vi "CompleteResourceUtilizationWithIFw.vi"() -> ()   [LabVIEW 2015]
uses:
  <instrlib>/_niInstr/PIO Register Bus/v0/Common/Command From Host.ctl
  <vilib>/Platform/TimedLoop/XDataNode/timing_clust.ctl
  <vilib>/Platform/TimedLoop/XDataNode/nitl_modes.ctl
  <vilib>/Platform/TimedLoop/XDataNode/wakeup.ctl
  <vilib>/rvi/Emulation/niFpgaGetClockAttributes.vi
  <vilib>/rvi/Emulation/niFpgaSctlEmulationGetInTimedLoop.vi
  <vilib>/rvi/Emulation/niFpgaEmulationReportErrorSimple.vi
  <vilib>/rvi/eio/common/nirviEmuTemplateMethod_errors.vi
  <vilib>/rvi/Emulation/niFpgaCriticalErrorInLSC.vi
  <vilib>/rvi/Emulation/niFpgaProcessEmulError.vi
  <vilib>/eio/EIONode/EIONode.xnode
  <vilib>/Platform/TimedLoop/XDataNode/XDataNode.xnode
  <instrlib>/_niInstr/Instruction Framework/v1/FPGA/Top Level Bus/Register Configuration/Register Configuration.lvclass
  <vilib>/Platform/TimedLoop/XDataNode/XDNodeRunTimeDep.lvlib
  ScaleAndLimit.lvlib
  AddressSpace.lvclass
  <instrlib>/_niInstr/PIO Register Bus/v0/FPGA/niInstr PIO Register Bus v0 FPGA.lvclass
  <instrlib>/_niInstr/PIO Register Bus/v0/Common/PIO Register Bus v0 Common.lvlib
panel:
  in  "fifo reg bus ctrl 0":u32
  out "fifo reg bus status 0":u32
  out "fifo reg bus data 0":u64
  in  "command":T1
  out "SimultaneousAILoopRate":u32
  out "ScaledAI":sgl[](array[numeric])
  # "Device Utilization\n---------------------------\nTotal Slices: 38.3% (5094 out of 13300)\nSlice Registers: 13.5% (14411 out of 106400)\nSlice LUTs: 24.6% (13093 out of 53200)\nBlock RAMs: 2.9% (4 out of 140)\nDSP48s: 1.4% (3 out of 220)"
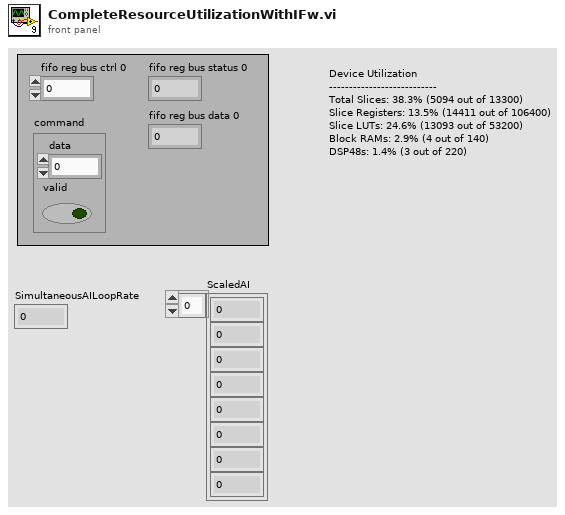
[diagram p1: front panel]
types:
  T1 = typedef "PIO Register Bus v0 Common.lvlib/Command From Host.ctl" = cluster{"data":u64, "valid":bool}
  T2 = typedef "XDNodeRunTimeDep.lvlib/timing_clust.ctl" = cluster{"Expected End [f-1]":u64, "Actual End [f-1]":u64, "Finished Late? [f-1]":bool, "Expected End [i-1]":u64, "Actual End [i-1]":u64, "Finished Late? [i-1]":bool, "Expected Start [i]":u64, "Actual Start [i]":u64, "Expected Start [f]":u64, "Actual Start [f]":u64, "Source Name":string, "Structure Name":string, "Period":i64, "Deadline":i64, "Offset":i64, "Start":i64, "Priority":i32, "Timeout":i32, "Mode":T3, "Wakeup Reason":T4, "Error":errorcluster, "Source Type":string, "Secondary Source Type":string, "Global End Time":u64, "Global Start Time":u64, "Frame Duration":u64, "Iteration Duration":u64, "Assigned CPU":i32, "I/O Scan Engine Mode":u32}
  T3 = typedef "XDNodeRunTimeDep.lvlib/nitl_modes.ctl" = enum32{"No Change", "Process missed periods, maintain original phase", "Discard missed periods, maintain original phase", "Process missed periods, ignore original phase", "Discard missed periods, ignore original phase"}
  T4 = typedef "XDNodeRunTimeDep.lvlib/wakeup.ctl" = enum32{"Normal", "Aborted", "Asynchronous wakeup", "Timing source error", "Timed loop error", "Timeout"}
  T5 = typedef "ScaleAndLimit.lvlib/LimitsRegisters.ctl" = cluster{"HighLimits":refnum<k21>, "LowLimits":refnum<k21>, "ClearLimits":refnum<k21>, "LimitsFlag":refnum<k21>}
  T6 = typedef "ScaleAndLimit.lvlib/ConfigRegisters.ctl" = cluster{"LimitsEnabled":refnum<k21>, "UnscaledHighLimit":refnum<k21>, "UnscaledLowLimit":refnum<k21>, "B":refnum<k21>, "M":refnum<k21>}
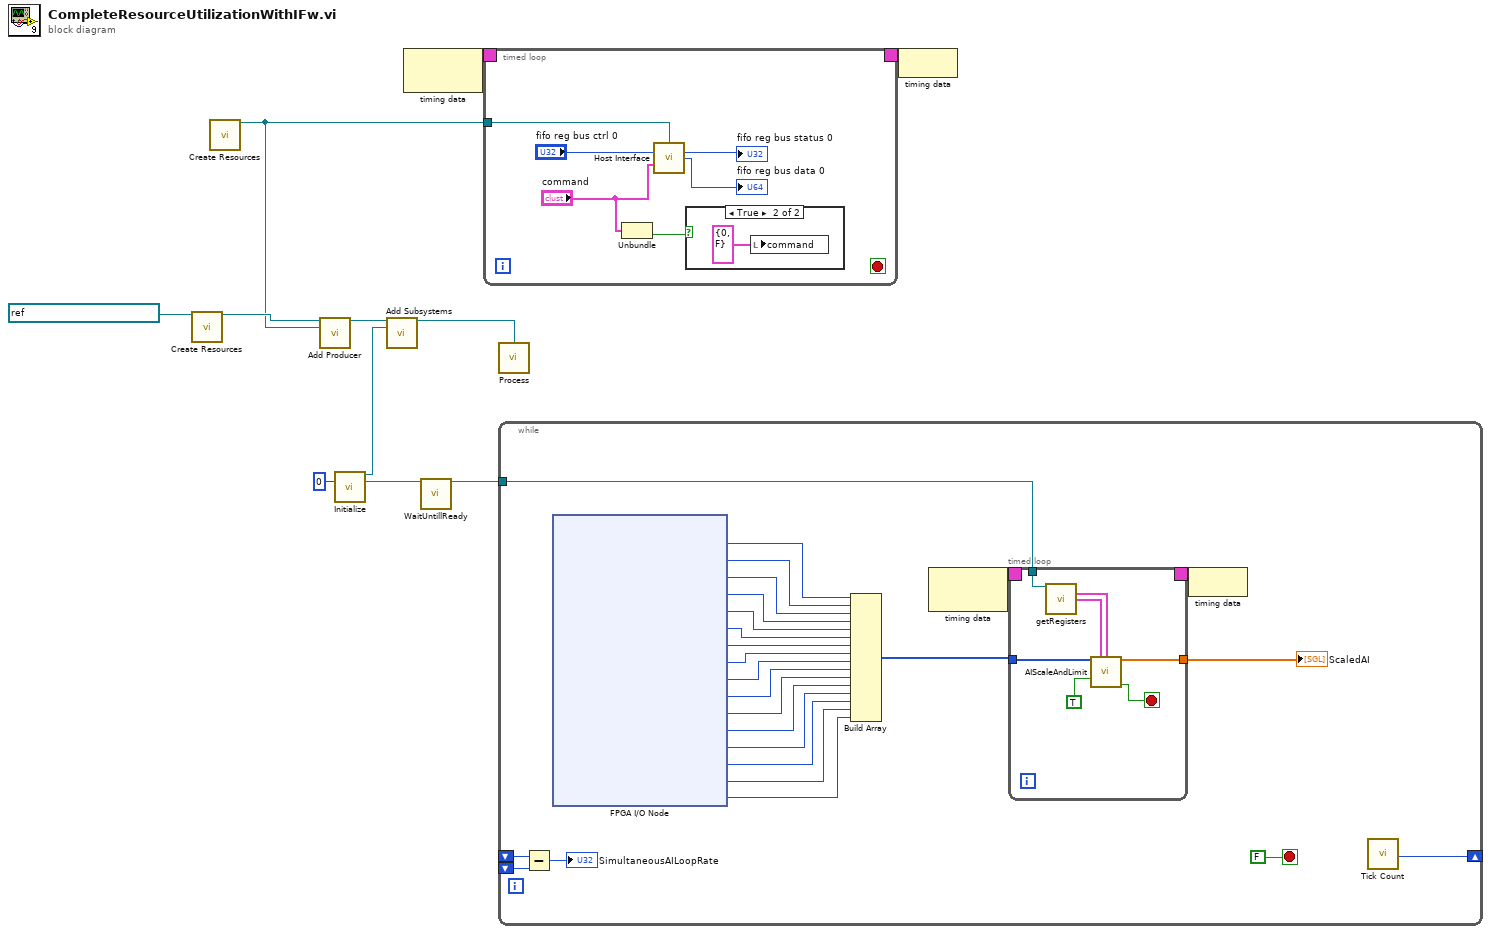
[diagram p0: block diagram]
diagram:
  n1 = call <instrlib>:"Create Resources.vi"("register clock"=refnum<k21> "40 MHz Onboard Clock") -> ("register configuration"=w9:refnum<class "Register Configuration.lvclass">)  [unwired: 14 in]
  n2 = call <instrlib>:"Create Resources.vi"() -> ("fifo register bus"=w1:refnum<class "niInstr PIO Register Bus v0 FPGA.lvclass">)  [unwired: 15 in]
  n3 = call <instrlib>:"Add Producer.vi"("register configuration in"=w9, "instruction producer"=w1) -> ("register configuration out"=w7:refnum<class "Register Configuration.lvclass">)  [unwired: 13 in]
  n4 = call "Initialize.vi"("instance"=u8 0) -> ("subsystem"=w6:refnum<class "Single Address Space Collection.lvclass">, "AddressSpace"=w3:refnum<class "AddressSpace.lvclass">)  [unwired: 13 in]
  n5 = call <instrlib>:"Add Subsystems.vi"("register configuration in"=w7, "subsystems"=w6) -> ("register configuration out"=w4:refnum<class "Register Configuration.lvclass">)  [unwired: 13 in]
  n6 = node-c288() -> (w11:T2)  [unwired: 1 in]
  n7 = call "WaitUntillReady.vi"("AddressSpace in"=w3) -> ("AddressSpace out"=w2:refnum<class "AddressSpace.lvclass">)  [unwired: 14 in]
  n8 = timed-loop {
    timing: w11 -> [_]
    timing-out: [_] -> w10
    tunnel: w1 -> [w16]
    stop <- _ stop-if-true
    n9 = Unbundle("command") -> ("valid"=w12:bool)  [unwired: 1 out]
    n10 = call <instrlib>:"Host Interface.vi"("fifo register bus"=w16, "fifo reg bus ctrl 0"="fifo reg bus ctrl 0", "command"="command") -> ("fifo reg bus status 0"=→"fifo reg bus status 0":u32, "fifo reg bus data 0"=→"fifo reg bus data 0":u64)  [unwired: 11 in]
    n11 = case shown="True" w12 {
      frame False {
      }
      frame True {
        n12 = local write "command"(T1 {"data"=0, "valid"=FALSE} ("command")) -> ()
      }
    }
  }
  n13 = call <instrlib>:"Process.vi"("register configuration"=w4) -> ()  [unwired: 15 in]
  n14 = while {
    shift-right: [w45] -> _
    shift-left: _ -> [w44]
    shift-left: _ -> [w43]
    tunnel: w2 -> [w23]
    stop <- FALSE stop-if-true
    n15 = Subtract(x=w44, y=w43) -> (x-y=→"SimultaneousAILoopRate":u32)
    n16 = xnode "FPGA I/O Node"() -> ("RMC/Simultaneous/AI0"=w41:i16, "RMC/Simultaneous/AI1"=w40:i16, "RMC/Simultaneous/AI2"=w39:i16, "RMC/Simultaneous/AI3"=w38:i16, "RMC/Simultaneous/AI4"=w37:i16, "RMC/Simultaneous/AI5"=w36:i16, "RMC/Simultaneous/AI6"=w35:i16, "RMC/Simultaneous/AI7"=w34:i16, "RMC/Simultaneous/AI8"=w33:i16, "RMC/Simultaneous/AI9"=w32:i16, "RMC/Simultaneous/AI10"=w31:i16, "RMC/Simultaneous/AI11"=w30:i16, "RMC/Simultaneous/AI12"=w29:i16, "RMC/Simultaneous/AI13"=w28:i16, "RMC/Simultaneous/AI14"=w27:i16, "RMC/Simultaneous/AI15"=w21:i16)  [unwired: 16 in, 16 out]
    n17 = Build Array(w41, w40, w39, w38, w37, w36, w35, w34, w33, w32, w31, w30, w29, w28, w27, w21) -> (w22:i16[])
    n18 = node-c288() -> (w26:T2)  [unwired: 1 in]
    n19 = timed-loop {
      timing: w26 -> [_]
      timing-out: [_] -> w25
      tunnel: w22 -> [w53]
      tunnel: [w51] -> w24
      tunnel: w23 -> [w49]
      stop <- w50 stop-if-true
      n20 = call "getRegisters.vi"("AddressSpace in"=w49) -> ("LimitsRegisters"=w48:T5, "ConfigRegisters"=w47:T6)  [unwired: 12 in, 1 out]
      n21 = call "AIScaleAndLimit.vi"("UnscaledAI"=w53, "ConfigRegisters"=w47, "LimitsRegisters"=w48, "input valid"=TRUE) -> ("ScaledAI"=w51:sgl[], "output valid"=w50:bool)  [unwired: 9 in, 1 out]
    }
    "ScaledAI" <- w24
    n22 = node-c288(w25) -> ()
    n23 = call "Tick Count"() -> ("Tick Count(Ticks)"=w45:u32)
  }
  n24 = node-c288(w10) -> ()
